vi "Receive from CS.vi"(8 "error in (no error)":errorcluster, 11 "TCS in":refnum<class "TCS.lvclass">) -> (0 "error out":errorcluster, 2 "Response string":string, 3 "TCS out":refnum<class "TCS.lvclass">)   [LabVIEW 2013, in "TCS.lvclass"]
uses:
  Lib.llb/TCS.lvclass
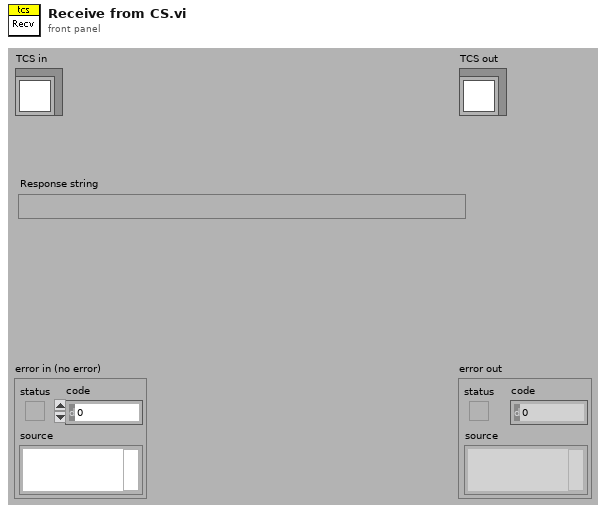
[diagram p1: front panel]
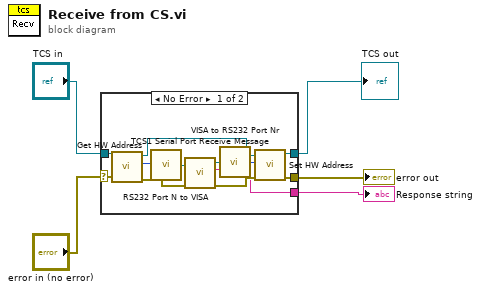
[diagram p0: block diagram]
diagram:
  n1 = case shown="No Error" "error in (no error)" {
    selector: "error in (no error)" -> [w16 w18]
    tunnel: [w12 w18] -> w5
    tunnel: [w11 _] -> w4
    tunnel: [w10 w19] -> w3
    tunnel: "TCS in" -> [w17 w19]
    frame No Error {
      n2 = call-dynamic "Get HW Address.vi"("error in (no error)"=w16, "CS.lvclass in"=w17) -> ("error out"=w14:errorcluster, "HW Address"=w9:u32, "CS.lvclass out"=w15:refnum<class "TCS.lvclass">)  [unwired: 7 in]
      n3 = call "RS232 Port N to VISA.vi"("Port Number"=w9) -> ("VISA Resource Name"=w8:refnum<visa-resource-name>)  [unwired: 1 in]
      n4 = call "TCS1 Serial Port Receive Message.vi"("TCS port"=w8, "error in"=w14) -> ("TCS port out"=w7:refnum<visa-resource-name>, "read buffer"=w11:string, "error out"=w13:errorcluster)  [unwired: 4 in, 1 out]
      n5 = call "VISA to RS232 Port Nr.vi"("VISA Resource Name"=w7) -> ("Port Number"=w6:u8)  [unwired: 1 in]
      n6 = call-dynamic "Set HW Address.vi"("error in (no error)"=w13, "HW Address"=w6, "CS.lvclass in"=w15) -> ("error out"=w12:errorcluster, "CS.lvclass out"=w10:refnum<class "TCS.lvclass">)  [unwired: 7 in]
    }
    frame Error {
    }
  }
  "error out" <- w5
  "TCS out" <- w3
  "Response string" <- w4
